vi "MGCC_OnliTopoIden.vi"() -> ()   [LabVIEW 2016]
doc: "-----------------------------------------------------------------------------------------------------------------------\nCopyright <2019> <The University of Tennessee at Knoxville and the University of Tennessee Research Foundation>\nThis software is released under BSD-3 \nhttps://opensource.org/licenses/BSD-3-Clause \nAdditional license options available at https://utrf.tennessee.edu/industry/sample-agreements/\n-----------------------------------------------------------------------------------------------------------------------\n\nSimplified version of topology identification, without support for dynamic boundary"
uses:
  Communication/Global communication.vi
  Model Management/Global_MdlMgmt.vi
  Communication/Global communication output.vi
  <vilib>/ErrorRing/Error Ring.xnode
panel:
  out "To Topology Identification":dbl[][](array[numeric])
  out "Microgrid Topology":dbl[][](array[numeric])
  in  "array":i16[](array[numeric])
  out "Status":dbl[](array[numeric])
  in  "element 2":dbl
  in  "element":dbl
  in  "B2":bool
  out "Island_status":bool
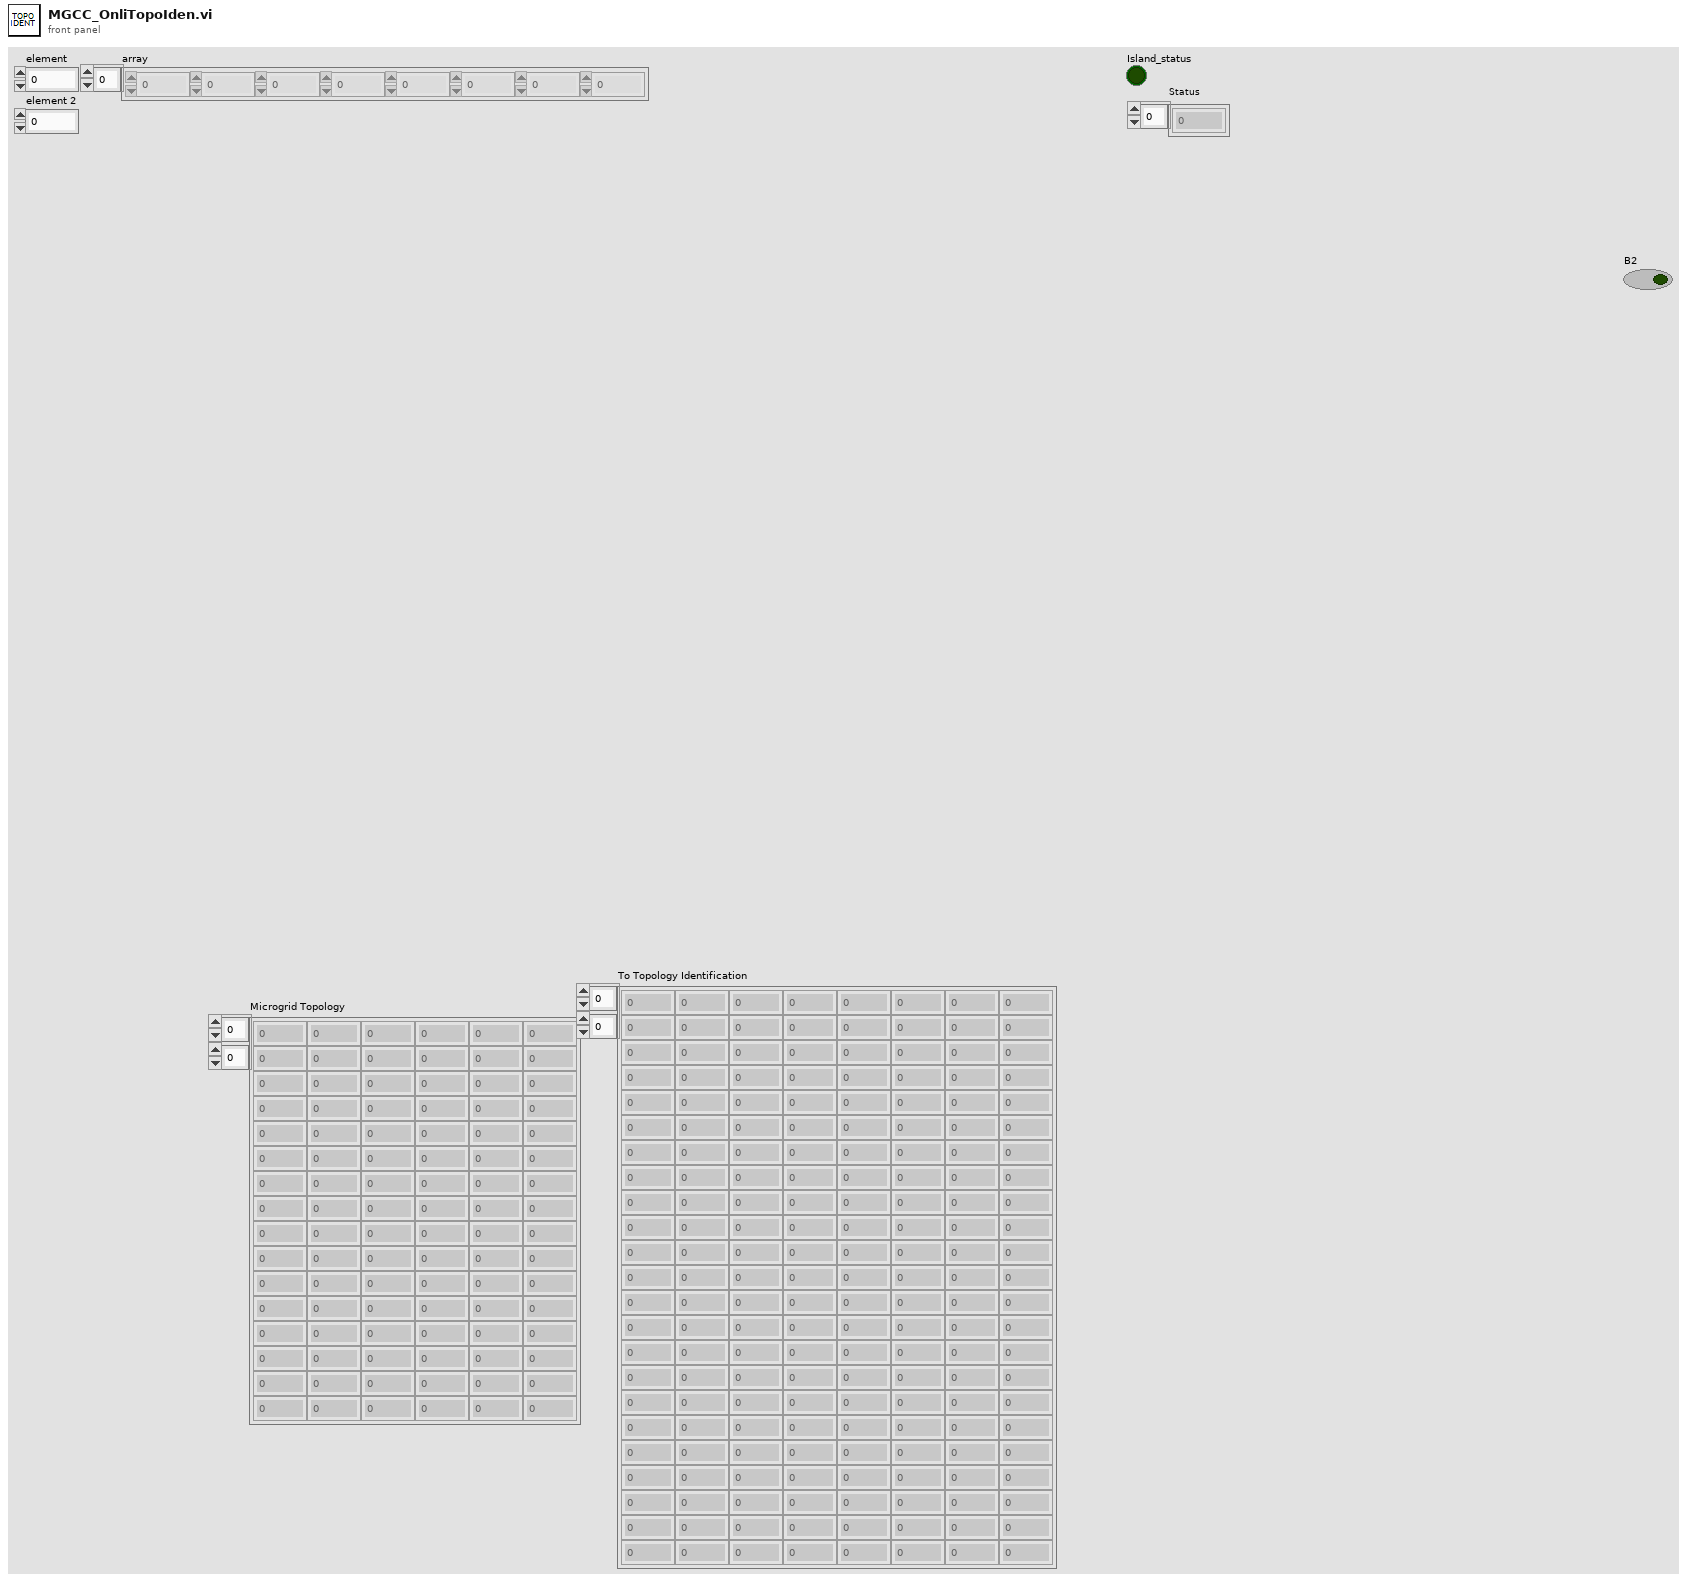
[diagram p1: front panel]
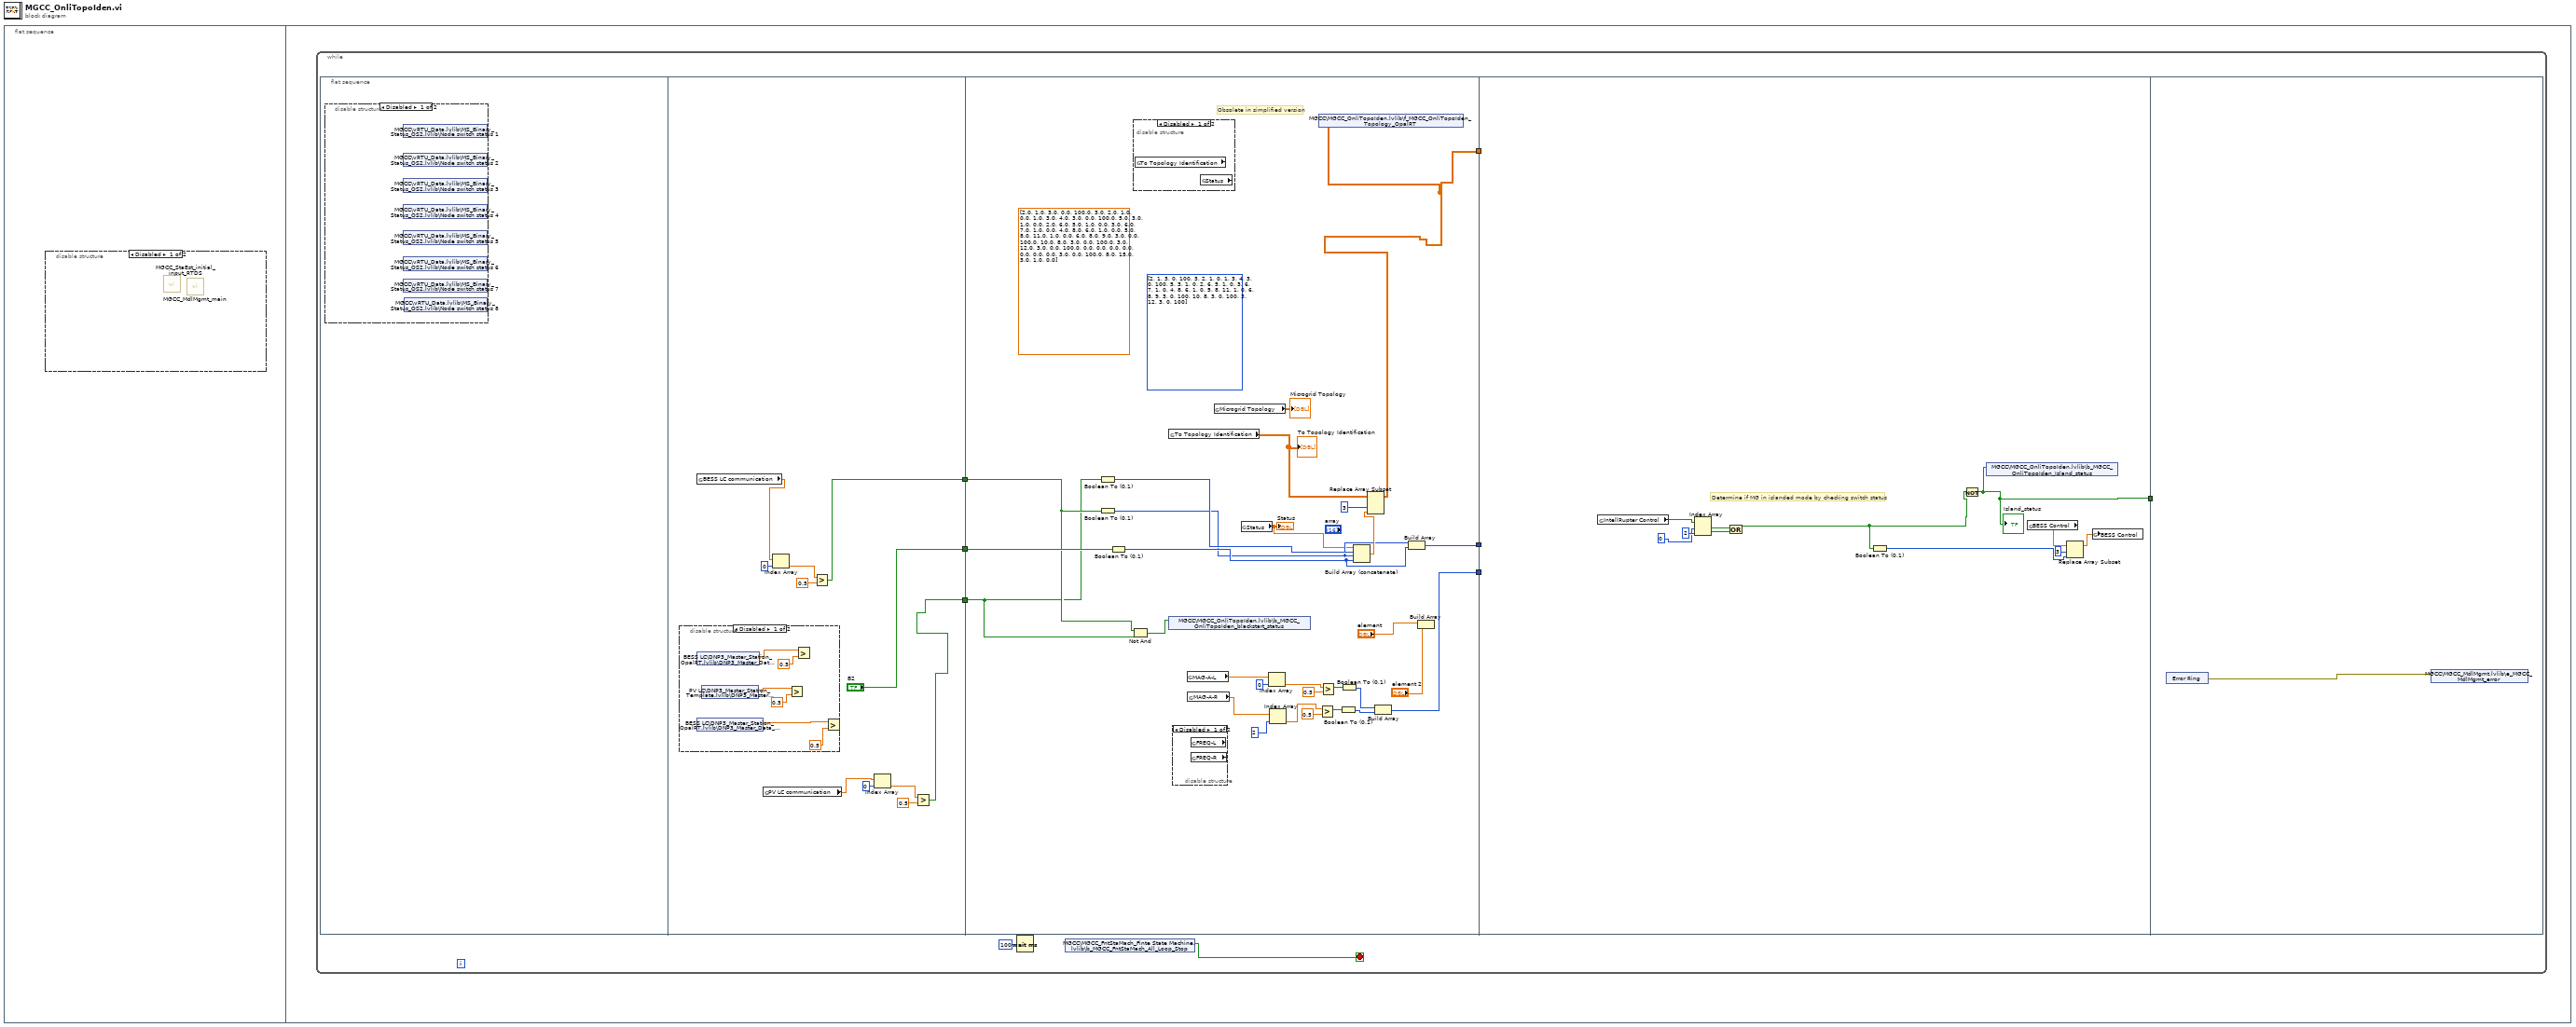
[diagram p0: block diagram]
diagram:
  n1 = flat-sequence {
    frame #0 {
      n2 = disable-structure shown="Disabled" {
        frame Disabled {
          n3 = call "MGCC_StaEst_initial_input_RTDS.vi"() -> ()  [unwired: 12 in]
          n4 = call "MGCC_MdlMgmt_main.vi"() -> ()  [unwired: 12 in]
        }
        frame Enabled {
        }
      }
    }
    frame #1 {
      n5 = while {
        stop <- w5 stop-if-true
        n6 = flat-sequence {
          tunnel: [w18] -> w8
          tunnel: [w24] -> w7
          tunnel: ["B2"] -> w3
          tunnel: w8 -> [w59]
          tunnel: w7 -> [w60]
          tunnel: [w57] -> w6
          tunnel: w3 -> [w62]
          tunnel: [w53] -> w2
          tunnel: [w37] -> w1
          tunnel: w6 -> [_]
          tunnel: [w74] -> w4
          tunnel: w2 -> [_]
          tunnel: w1 -> [_]
          tunnel: w4 -> [_]
          frame #0 {
            n7 = disable-structure shown="Disabled" {
              frame Disabled {
                n8 = shared-variable "MGCC\\vRTU_Data.lvlib\\MS_Binary_Status_OS2.lvlib\\Node switch status 1"() -> (w17:bool)  [unwired: 1 in, 1 out]
                n9 = shared-variable "MGCC\\vRTU_Data.lvlib\\MS_Binary_Status_OS2.lvlib\\Node switch status 2"() -> (w16:bool)  [unwired: 1 in, 1 out]
                n10 = shared-variable "MGCC\\vRTU_Data.lvlib\\MS_Binary_Status_OS2.lvlib\\Node switch status 3"() -> (w15:bool)  [unwired: 1 in, 1 out]
                n11 = shared-variable "MGCC\\vRTU_Data.lvlib\\MS_Binary_Status_OS2.lvlib\\Node switch status 4"() -> (w14:bool)  [unwired: 1 in, 1 out]
                n12 = shared-variable "MGCC\\vRTU_Data.lvlib\\MS_Binary_Status_OS2.lvlib\\Node switch status 5"() -> (w13:bool)  [unwired: 1 in, 1 out]
                n13 = shared-variable "MGCC\\vRTU_Data.lvlib\\MS_Binary_Status_OS2.lvlib\\Node switch status 6"() -> (w12:bool)  [unwired: 1 in, 1 out]
                n14 = shared-variable "MGCC\\vRTU_Data.lvlib\\MS_Binary_Status_OS2.lvlib\\Node switch status 7"() -> (w11:bool)  [unwired: 1 in, 1 out]
                n15 = shared-variable "MGCC\\vRTU_Data.lvlib\\MS_Binary_Status_OS2.lvlib\\Node switch status 8"() -> (w10:bool)  [unwired: 1 in, 1 out]
              }
              frame Enabled {
              }
            }
          }
          frame #1 {
            n16 = disable-structure shown="Disabled" {
              frame Disabled {
                n17 = shared-variable "BESS LC\\DNP3_Master_Station_OpalRT.lvlib\\DNP3_Master_Data_Variables.lvlib\\MS_Analog_Status.lvlib\\BESS-STATUS"() -> (w32:dbl)  [unwired: 1 in, 1 out]
                n18 = shared-variable "BESS LC\\DNP3_Master_Station_OpalRT.lvlib\\DNP3_Master_Data_Variables.lvlib\\MS_Analog_Status.lvlib\\BESS2-STATUS"() -> (w29:dbl)  [unwired: 1 in, 1 out]
                n19 = shared-variable "PV LC\\DNP3_Master_Station_Template.lvlib\\DNP3_Master_Data_Variables.lvlib\\MS_Analog_Status.lvlib\\PV-STATUS"() -> (w31:dbl)  [unwired: 1 in, 1 out]
                n20 = Greater?(x=w31, y=0.5) -> ()  [unwired: 1 out]
                n21 = Greater?(x=w32, y=0.5) -> ()  [unwired: 1 out]
                n22 = Greater?(x=w29, y=0.5) -> ()  [unwired: 1 out]
              }
              frame Enabled {
              }
            }
            n23 = global read "Global communication.vi" "BESS LC communication"() -> (w23:dbl[])
            n24 = global read "Global communication.vi" "PV LC communication"() -> (w19:dbl[])
            n25 = Index Array(array=w23, index=0) -> (element=w25:dbl)
            n26 = Greater?(x=w25, y=0.5) -> (0:w24:bool)
            n27 = Index Array(array=w19, index=0) -> (element=w20:dbl)
            n28 = Greater?(x=w20, y=0.5) -> (0:w18:bool)
          }
          frame #2 {
            (unwired) i32[][] [[2, 1, 3, 0, 100], [3, 2, 1, 0, 1], [3, 4, 3, 0, 100], [5, 3, 1, 0, 2], [6, 5, 1, 0, 3], [6, 7, 1, 0, 4], [8, 6, 1, 0, 5], [8, 11, 1, 0, 6], [8, 9, 3, 0, 100], [10, 8, 3, 0, 100], [3, 12, 3, 0, 100]]
            (unwired) dbl[][] [[2.0, 1.0, 3.0, 0.0, 100.0], [3.0, 2.0, 1.0, 0.0, 1.0], [3.0, 4.0, 3.0, 0.0, 100.0], [5.0, 3.0, 1.0, 0.0, 2.0], [6.0, 5.0, 1.0, 0.0, 3.0], [6.0, 7.0, 1.0, 0.0, 4.0], [8.0, 6.0, 1.0, 0.0, 5.0], [8.0, 11.0, 1.0, 0.0, 6.0], [8.0, 9.0, 3.0, 0.0, 100.0], [10.0, 8.0, 3.0, 0.0, 100.0], [3.0, 12.0, 3.0, 0.0, 100.0], [0.0, 0.0, 0.0, 0.0, 0.0], [0.0, 0.0, 3.0, 0.0, 100.0], [8.0, 15.0, 3.0, 1.0, 0.0]] ("f_MGCC_MdlMgmt_Topology_OpalRT")
            # "Obsolete in simplified version"
            n29 = Boolean To (0,1)(Boolean=w59) -> (0, 1=w56:i16)
            n30 = Boolean To (0,1)(Boolean=w60) -> (0, 1=w54:i16)
            n31 = Boolean To (0,1)(Boolean=w62) -> (0, 1=w55:i16)
            n32 = Not And(1:w59, 2:w60) -> (0:w63:bool)
            n33 = disable-structure shown="Disabled" {
              frame Disabled {
                n34 = global read "Global_MdlMgmt.vi" "To Topology Identification"() -> ()  [unwired: 1 out]
                n35 = global read "Global communication.vi" "Status"() -> ()  [unwired: 1 out]
              }
              frame Enabled {
              }
            }
            n36 = shared-variable "MGCC\\MGCC_OnliTopoIden.lvlib\\b_MGCC_OnliTopoIden_blackstart_status"(w63) -> ()  [unwired: 1 in, 1 out]
            n37 = global read "Global_MdlMgmt.vi" "To Topology Identification"() -> (w36:dbl[][])
            "To Topology Identification" <- w36
            n38 = disable-structure shown="Disabled" {
              frame Disabled {
                n39 = global read "Global communication.vi" "FREQ-L"() -> ()  [unwired: 1 out]
                n40 = global read "Global communication.vi" "FREQ-R"() -> ()  [unwired: 1 out]
              }
              frame Enabled {
              }
            }
            n41 = global read "Global communication.vi" "MAG-A-L"() -> (w49:dbl[])
            n42 = global read "Global communication.vi" "MAG-A-R"() -> (w40:dbl[])
            n43 = global read "Global_MdlMgmt.vi" "Microgrid Topology"() -> (→"Microgrid Topology":dbl[][])
            n44 = global read "Global communication.vi" "Status"() -> (w50:dbl[])
            "Status" <- w50
            n45 = Index Array(array=w49, index=0) -> (element=w46:dbl)
            n46 = Index Array(array=w40, index=2) -> (element=w38:dbl)
            n47 = Greater?(x=w38, y=0.5) -> (0:w44:bool)
            n48 = Greater?(x=w46, y=0.5) -> (0:w45:bool)
            n49 = Boolean To (0,1)(Boolean=w44) -> (0, 1=w41:i16)
            n50 = Boolean To (0,1)(Boolean=w45) -> (0, 1=w42:i16)
            n51 = Build Array (concatenate)(w50, w56, w54, w55) -> (w58:dbl[])
            n52 = Replace Array Subset(array=w36, new element=w58, index (col)=3 ("disabled index (col)")) -> (w57:dbl[][])  [unwired: 1 in]
            n53 = shared-variable "MGCC\\MGCC_OnliTopoIden.lvlib\\f_MGCC_OnliTopoIden_Topology_OpalRT"(w57) -> ()  [unwired: 1 in, 1 out]
            n54 = Build Array(w42, w41) -> (w37:i16[])
            n55 = Build Array(w54, w55) -> (w53:i16[])
            n56 = Build Array("element", "element 2") -> ()  [unwired: 1 out]
          }
          frame #3 {
            # "Determine if MG in islanded mode by checking switch status"
            n57 = global read "Global communication output.vi" "IntellRupter Control"() -> (w70:bool[])
            n58 = Index Array(array=w70, index #1=0 ("index"), index #2=2 ("index")) -> (element #1=w67:bool, element #2=w66:bool)
            n59 = Or(x=w67, y=w66) -> (x .or. y?=w65:bool)
            n60 = Boolean To (0,1)(Boolean=w65) -> (0, 1=w64:i16)
            n61 = Not(x=w65) -> (.not. x?=w74:bool)
            "Island_status" <- w74
            n62 = shared-variable "MGCC\\MGCC_OnliTopoIden.lvlib\\b_MGCC_OnliTopoIden_Island_status"(w74) -> ()  [unwired: 1 in, 1 out]
            n63 = global read "Global communication output.vi" "BESS Control"() -> (w73:dbl[])
            n64 = Replace Array Subset(array=w73, new element=w64, index=3) -> (w72:dbl[])
            n65 = global write "Global communication output.vi" "BESS Control"(w72) -> ()
          }
          frame #4 {
            n66 = xnode "Error Ring"() -> ("error out"=w75:errorcluster)
            n67 = shared-variable "MGCC\\MGCC_MdlMgmt.lvlib\\e_MGCC_MdlMgmt_error"(w75) -> ()  [unwired: 1 in, 1 out]
          }
        }
        n68 = Wait (ms)(milliseconds to wait=u32 100) -> ()  [unwired: 1 out]
        n69 = shared-variable "MGCC\\MGCC_FntStaMach_Finte State Machine.lvlib\\b_MGCC_FntStaMach_All_Loop_Stop"() -> (w5:bool)  [unwired: 1 in, 1 out]
      }
    }
  }
